vi "气象全局变量.vi"() -> ()   [LabVIEW 2016, in "AIRMAR WeatherCaster.lvlib"]
uses:
  AIRMAR WeatherCaster.lvlib
panel:
  in  "气象仪型号":enum16{"NMEA", "WXA100"}(ring)
  in  "数据库类型":T1
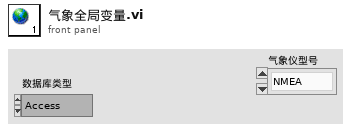
[diagram p1: front panel]
types:
  T1 = typedef "数据库类型.ctl" = enum16{"Access", "SQLite"}
diagram:
